vi "Receive Error.vi"(8 "error in":errorcluster, 10 "Receive Error":errorcluster, 11 "_Parent Actor Template in":refnum<class "_Parent Actor Template.lvclass">) -> (0 "error out":errorcluster, 3 "_Parent Actor Template out":refnum<class "_Parent Actor Template.lvclass">)   [LabVIEW 2016, in "_Parent Actor Template.lvlib" / "_Parent Actor Template.lvclass"]
uses:
  _Parent Actor Template.lvclass
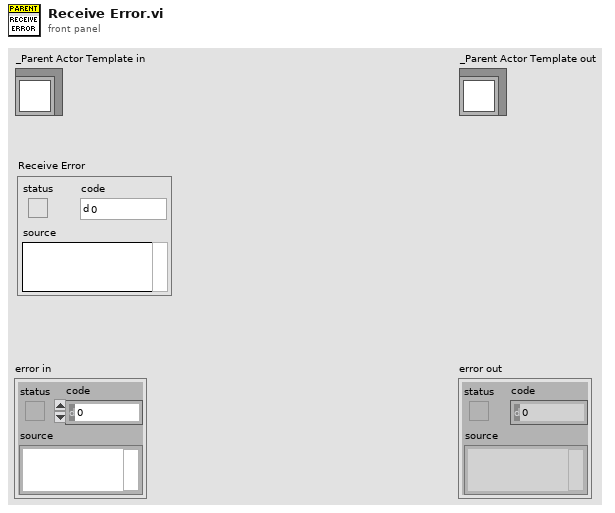
[diagram p1: front panel]
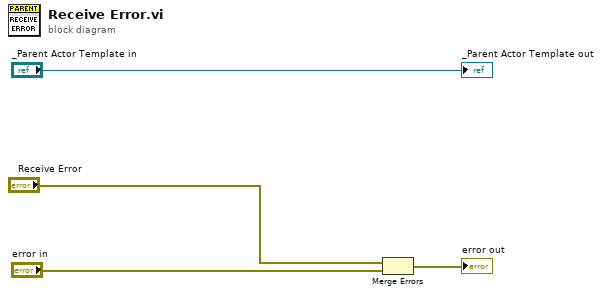
[diagram p0: block diagram]
diagram:
  n1 = Merge Errors("Receive Error", "error in") -> (→"error out":errorcluster)
  "_Parent Actor Template out" <- "_Parent Actor Template in"
